vi "Do.vi"(8 "error in":errorcluster, 10 "Actor in":refnum<class "Actor.lvclass">, 11 "Save Data MSG":refnum<class "Save Data MSG.lvclass">) -> (0 "error out":errorcluster, 2 "Actor out":refnum<class "Actor.lvclass">)   [LabVIEW 2014, in "Controller.lvlib" / "Save Data MSG.lvclass"]
doc: "(<B>Filename</B>: Actor Framework.lvlib:Message.lvclass:Do.vi)\n\nDefines what a message does when it is received by an actor. Generally, a message instructs an actor to invoke one of its methods. By default, this method does nothing. A child class must override it to define behavior. Create a child class by using the Actor Framework Message Maker dialog box."
uses:
  Save Data MSG.lvclass
  <vilib>/ActorFramework/Actor/Actor.lvclass
  Save Data MSG.lvclass/Save Data MSG.ctl
  File Actor/Messages/To/Save/Change File Writing State MSG.lvclass
  Controller.lvclass
  Controls/eMap.ctl
  <vilib>/ActorFramework/Message Enqueuer/Message Enqueuer.lvclass
  SuperActor/SuperActor.lvclass/SuperActor.ctl
  Controller.lvclass/Controller.ctl
  File Actor/Messages/To/Save/Change File Writing State MSG.lvclass/Change File Writing State MSG.ctl
  <vilib>/ActorFramework/Message Enqueuer/Message Enqueuer.lvclass/Message Enqueuer.ctl
  File Actor/Messages/To/Save/Write Save_.vi
  SuperActor/Read Log Session.vi
  SuperActor/Read CVT Session.vi
  Accessors/Read Enqueuer Map.vi
  <vilib>/ActorFramework/Message Priority Queue/Priority Enqueue.vi
  <userlib>/_Session Fwk/Session - Root.lvclass
  reusable/Session APIs/Session Log/System Log.lvclass
  reusable/Session APIs/CVT/CVT.lvclass
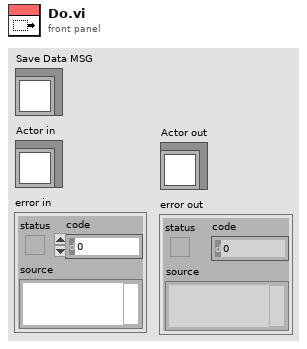
[diagram p1: front panel]
types:
  T1 = typedef "Controller.lvlib/Controller.lvclass/eMap.ctl" = cluster{"Enqueuer":refnum<class "Message Enqueuer.lvclass">, "Active":bool}
  T2 = typedef "Session - Root.lvclass/Session Handle.ctl" = refnum<data-value>
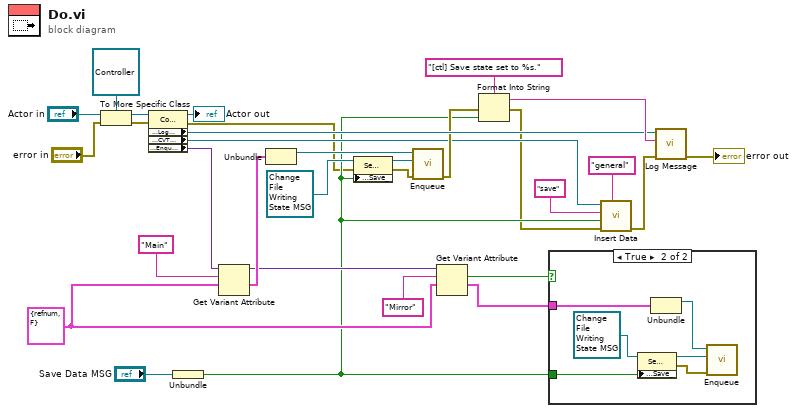
[diagram p0: block diagram]
diagram:
  w12 = T1 {"Enqueuer"=refnum, "Active"=FALSE} ("eMap")
  n1 = To More Specific Class(target class=refnum<class "Controller.lvclass"> refnum ("Controller.lvlib:Controller"), reference="Actor in", error in="error in") -> (specific class reference=w26:refnum<class "Controller.lvclass">, error out=w27:errorcluster)
  n2 = property class="Controller"(reference=w26, error in=w27) -> (reference out=→"Actor out":refnum<class "Controller.lvclass">, error out=w1:errorcluster, "Accessors:Log Session"=w20:T2, "Accessors:CVT Session"=w9:T2, "Accessors:Enqueuer Map"=w2:variant)
  n3 = Unbundle("Save Data MSG") -> (w6:bool)
  n4 = Get Variant Attribute(Variant=w2, name="Main", default value (empty Variant)=w12) -> (duplicate Variant=w11:variant, value=w18:T1)  [unwired: 1 in, 2 out]
  n5 = Unbundle(w18) -> ("Enqueuer"=w17:refnum<class "Message Enqueuer.lvclass">)  [unwired: 1 out]
  n6 = property class="Set File Save State"(reference=refnum<class "Change File Writing State MSG.lvclass"> refnum ("File Library.lvlib:Set File Save State"), error in=w1, "Accessors:Save_"=w6) -> (reference out=w24:refnum<class "Change File Writing State MSG.lvclass">, error out=w23:errorcluster)
  n7 = call <vilib>:"Enqueue.vi"("error in (no error)"=w23, "Message"=w24, "Message Enqueuer in"=w17) -> ("error out"=w15:errorcluster)  [unwired: 7 in, 1 out]
  n8 = Get Variant Attribute(Variant=w11, name="Mirror", default value (empty Variant)=w12) -> (found=w10:bool, value=w14:T1)  [unwired: 1 in, 2 out]
  n9 = Format Into String(format string="[ctl] Save state set to %s.", error in=w15, w6) -> (resulting string=w21:string, error out=w5:errorcluster)  [unwired: 1 in]
  n10 = case shown="True" w10 {
    tunnel: w14 -> [_ w37]
    tunnel: w6 -> [_ w32]
    frame False {
    }
    frame True {
      n11 = property class="Set File Save State"(reference=refnum<class "Change File Writing State MSG.lvclass"> refnum ("File Library.lvlib:Set File Save State"), "Accessors:Save_"=w32) -> (reference out=w35:refnum<class "Change File Writing State MSG.lvclass">, error out=w36:errorcluster)  [unwired: 1 in]
      n12 = Unbundle(w37) -> ("Enqueuer"=w33:refnum<class "Message Enqueuer.lvclass">)  [unwired: 1 out]
      n13 = call <vilib>:"Enqueue.vi"("error in (no error)"=w36, "Message"=w35, "Message Enqueuer in"=w33) -> ()  [unwired: 7 in, 2 out]
    }
  }
  n14 = call "Insert Data.vi"("Group"="general", "error in"=w5, "Data"=w6, "tag"="save", "CVT Session In"=w9) -> ("error out"=w4:errorcluster)  [unwired: 5 in, 1 out]
  n15 = call "Log Message.vi"("error in"=w4, "MSG In"=w21, "session in"=w20) -> ("error out"=→"error out":errorcluster)  [unwired: 7 in, 1 out]
